vi "launch custom VI.vi"(10 "messageHandler in":T2 {"params"."controlChannels"."ballControl" items=["Module6/output0", "Module6/output1", "Module6/output2", "Module6/output3", "Not-Used"]; "params"."controlChannels"."butterflyControl" items=["Module6/output0", "Module6/output1", "Module6/output2", "Module6/output3", "Not-Used"]; "params"."controlChannels"."speedControl" items=["Module6/output0", "Module6/output1", "Module6/output2", "Module6/output3", "Not-Used"]}, 11 "Queues in":T1) -> (3 "messageHandler out":T2 {"params"."controlChannels"."ballControl" items=["Module6/output0", "Module6/output1", "Module6/output2", "Module6/output3", "Not-Used"]; "params"."controlChannels"."butterflyControl" items=["Module6/output0", "Module6/output1", "Module6/output2", "Module6/output3", "Not-Used"]; "params"."controlChannels"."speedControl" items=["Module6/output0", "Module6/output1", "Module6/output2", "Module6/output3", "Not-Used"]})   [LabVIEW 2018]
uses:
  type defs/message handler data.ctl
  customVI/liveData/state.ctl
  type defs/Queues.ctl
  ICL-LabVIEW_General/Message Scheduler/generic message queue/standard message queue/standard message.lvclass
  <vilib>/Utility/error.llb/Error Cluster From Error Code.vi
  ICL-LabVIEW_General/data channels/parent class/Supporting functions/channel filter - active.vi
  supporting VIs/polymorphic VIs/enqueue for comms.vi
  <vilib>/ErrorRing/Error Ring.xnode
  ICL-LabVIEW_General/data channels/data channels.lvlib
types:
  T1 = typedef "Queues.ctl" = cluster{"messageHandler":refnum<queue>, "comms":refnum<queue>, "dataStream":refnum<queue>, "dataProcessor":refnum<queue>, "fileIO":refnum<queue>, "userInterface":refnum<queue>, "errors":refnum<queue>, "customCompressor":refnum<queue>}
  T2 = typedef "message handler data.ctl" = cluster{"params":cluster{"configFileID":u32, "configFilePath":path, "channelConfigFilePath":path, "incidentLogfile":path, "controlChannels":cluster{"ballControl":u16, "butterflyControl":u16, "speedControl":u16}, "pulsatorVIPath":path, "customVIPath":path, "HowdenAir":cluster{"vent Howden":bool, "Howden%":dbl}}, "vars":cluster{"commsStatus":bool[], "controlIndex":cluster{"ballControl":u16, "butterflyControl":u16, "speedControl":u16}, "customVIRef":refnum<vi>, "Interlocks":cluster{"gearboxOil":bool, "bearingOil":bool, "gearboxAir":bool}, "motorRunning":bool, "liveDataQ":refnum<queue>[]}}
  T3 = cluster{"standard message out":refnum<class "standard message.lvclass">, "ms delay":u32}
  T4 = typedef "channelControl.ctl" = cluster{"index":u16, "active":bool, "channelType":T5, "module":u16, "terminal":u16, "channelName":string, "scalingMethod":T6, "scalingParameters":dbl[], "scaledUnits":string, "tempOffset":dbl}
  T5 = typedef "channelScalingTypes.ctl" = enum16{"calculation", "measurement", "scanivalve", "output", "digital"}
  T6 = typedef "scalingMethods.ctl" = enum16{"none", "linear", "thermocouple", "polynomial", "encoder", "RTD"}
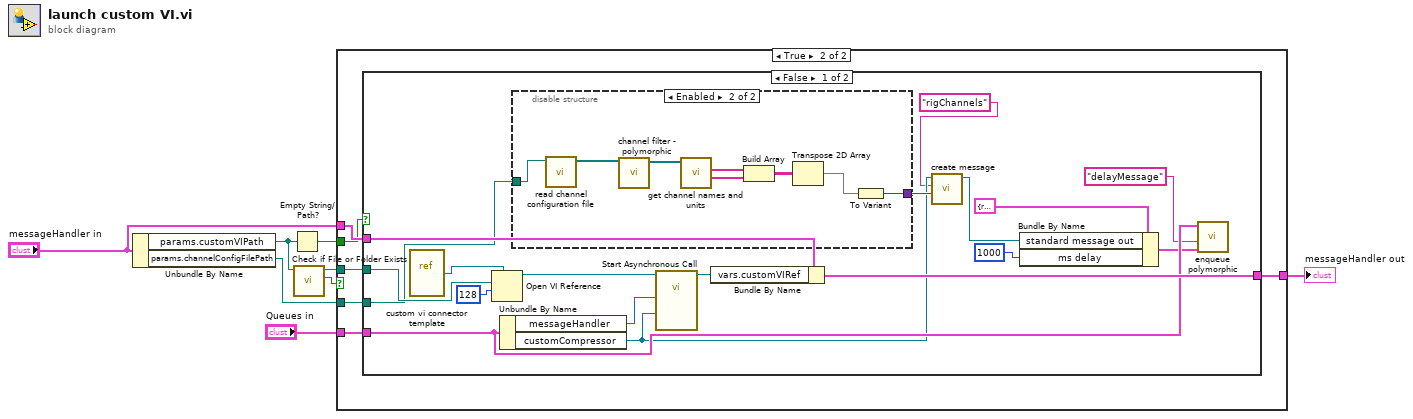
[diagram p0: block diagram]
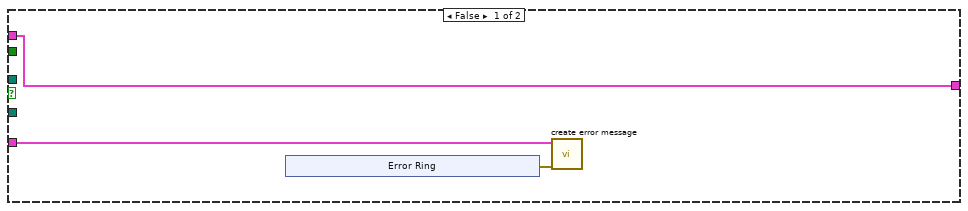
[diagram p2: hidden frame]
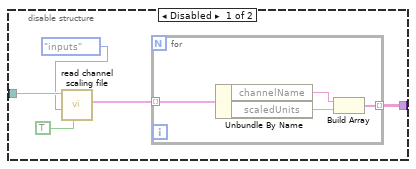
[diagram p3: hidden frame]
diagram:
  n1 = Unbundle By Name("messageHandler in") -> ("params.customVIPath"=w3:path, "params.channelConfigFilePath"=w4:path)
  n2 = Empty String/Path?(string/path=w3) -> (empty?=w5:bool)
  n3 = call <vilib>:"Check if File or Folder Exists.vi"("path"=w3) -> ("file or folder exists?"=w1:bool, "dup path"=w2:path)  [unwired: 8 in, 1 out]
  n4 = case shown="True" w1 {
    tunnel: [w11 w22] -> w8
    tunnel: "messageHandler in" -> [w11 w21]
    tunnel: "Queues in" -> [w10 w20]
    tunnel: w5 -> [_ w19]
    tunnel: w4 -> [_ w18]
    tunnel: w2 -> [_ w17]
    frame False {
      n5 = xnode "Error Ring"() -> ("error out"=w9:errorcluster)
      n6 = call "create error message.vi"("error in (no error)"=w9, "queues"=w10) -> ()  [unwired: 10 in]
    }
    frame True {
      n7 = case shown="False" w19 {
        tunnel: w17 -> [w40 _]
        tunnel: w20 -> [w32 _]
        tunnel: [w35 w58] -> w22
        tunnel: w21 -> [w36 w58]
        tunnel: w18 -> [w33 _]
        frame False {
          n8 = vi-ref "custom vi connector template.vi"() -> (w37:refnum<vi>)
          n9 = Open VI Reference(type specifier VI Refnum (for type only)=w37, vi path=w40, options=128) -> (vi reference=w38:refnum<vi>)  [unwired: 3 in, 1 out]
          n10 = Unbundle By Name(w32) -> ("messageHandler"=w25:refnum<queue>, "customCompressor"=w24:refnum<queue>)
          n11 = disable-structure shown="Enabled" {
            disable-tunnel: w33 -> [w45 w57]
            disable-tunnel: [w43 w50] -> w30
            frame Disabled {
              n12 = call "read channel scaling file.vi"("suppress inactive? (F)"=TRUE, "mode (all)"=enum16{"all", "inputs", "outputs", "digital"}."inputs", "file path"=w45) -> ("channelConfig"=w44:T4[])  [unwired: 4 in, 4 out]
              n13 = for {
                tunnel: w44 -> [w49] mode=indexing
                tunnel: [w46] -> w43 mode=indexing
                n14 = Unbundle By Name(w49) -> ("channelName"=w48:string, "scaledUnits"=w47:string)
                n15 = Build Array(w48, w47) -> (w46:string[])
              }
            }
            frame Enabled {
              n16 = call "read channel configuration file.vi"("config file"=w57) -> ("channelsArray"=w56:refnum<class "Data Channel.lvclass">[])  [unwired: 8 in, 2 out]
              n17 = call-poly "channel filter - polymorphic.vi"("channels"=w56) -> ("activeChannels"=w55:refnum<class "Data Channel.lvclass">[])  [unwired: 9 in, 1 out]
              n18 = call "get channel names and units.vi"("channels"=w55) -> ("channelUnits"=w53:string[], "channelName"=w54:string[])  [unwired: 7 in, 2 out]
              n19 = Build Array(w54, w53) -> (w52:string[][])
              n20 = Transpose 2D Array(2D array=w52) -> (transposed array=w51:string[][])
              n21 = To Variant(anything=w51) -> (Variant=w50:variant)
            }
          }
          n22 = call-by-ref "Start Asynchronous Call"(reference=w38, "customQueue"=w24, "parentQueue"=w25) -> (reference out=w34:refnum<vi>)  [unwired: 11 in, 1 out]
          n23 = Bundle By Name(cluster=w36, "vars.customVIRef"=w34) -> (w35:T2)
          n24 = call "create message.vi"("data"=w30, "message"="rigChannels", "queue ref"=w24) -> ("standard message out"=w28:refnum<class "standard message.lvclass">)  [unwired: 7 in, 1 out]
          n25 = Bundle By Name(cluster=T3 {"standard message out"=refnum, "ms delay"=1000}, "standard message out"=w28, "ms delay"=u32 1000) -> (w26:T3)
          n26 = call-poly "enqueue polymorphic.vi"("data"=w26, "message"="delayMessage", "Queues"=w32) -> ()  [unwired: 8 in, 1 out]
        }
        frame True {
        }
      }
    }
  }
  "messageHandler out" <- w8
